vi "ASI Get Video Data.vi"(7 "iWaitms":i32, 9 "lBuffSize":i32, 11 "iCameraID":i32) -> (0 "pBuffer out":u8[](array[numeric]), 3 "function return":i32)   [LabVIEW 2012, in "ASICamera2_no_err.lvlib"]
doc: "ASICAMERA_API ASI_ERROR_CODE ASIGetVideoData(int iCameraID, unsigned char* pBuffer, long lBuffSize, int iWaitms);"
uses:
  <userlib>/ASICamera2_no_err/ASICamera2_no_err.lvlib
  ASICamera2.dll
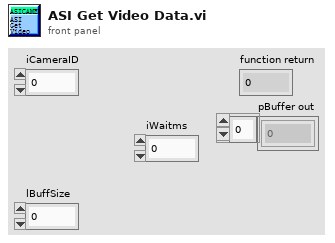
[diagram p1: front panel]
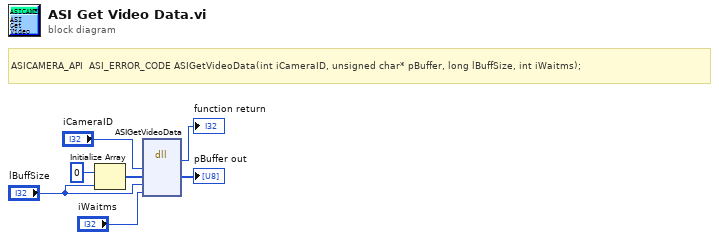
[diagram p0: block diagram]
diagram:
  # "ASICAMERA_API  ASI_ERROR_CODE ASIGetVideoData(int iCameraID, unsigned char* pBuffer, long lBuffSize, int iWaitms);"
  n1 = Initialize Array(u8 0, "lBuffSize") -> (w1:u8[])
  n2 = dll-call lib="ASICamera2.*" fn="ASIGetVideoData"("iCameraID"="iCameraID", "pBuffer"=w1, "lBuffSize"="lBuffSize", "iWaitms"="iWaitms") -> ("返回类型"=→"function return":i32, "pBuffer"=→"pBuffer out":u8[])  [unwired: 6 in, 2 out]
